vi "Install latest RSS and all addons.vi"(7 "restart automatically (T)":bool=TRUE, 8 "error in (no error)":errorcluster, 10 "Repository Location":string="\\\\uto-m34-1\\c$\\Program Files (x86)\\National Instruments\\RT Images", 11 "RT Management in":refnum<class "RT Management.lvclass">) -> (0 "error out":errorcluster, 2 "broken dependencies":T1[](array[typedef]) {"dependee"."component type" items=["standard", "hidden", "system", "unknown", "startup"]; "depender"."component type" items=["standard", "hidden", "system", "unknown", "startup"]}, 3 "RT Management out":refnum<class "RT Management.lvclass">)   [LabVIEW 2015, in "RT Management.lvlib" / "RT Management.lvclass"]
uses:
  RT Management.lvclass
  <vilib>/nisyscfg/Broken Dependency 1.2.ctl
  <vilib>/nisyscfg/Software 1.2.ctl
  <vilib>/nisyscfg/Component Type.ctl
  RT Management.lvclass/RT Management.ctl
  Get SysCfg Session.vi
  <vilib>/nisyscfg/Install Set.vi
  <vilib>/nisyscfg/nisyscfg.lvlib
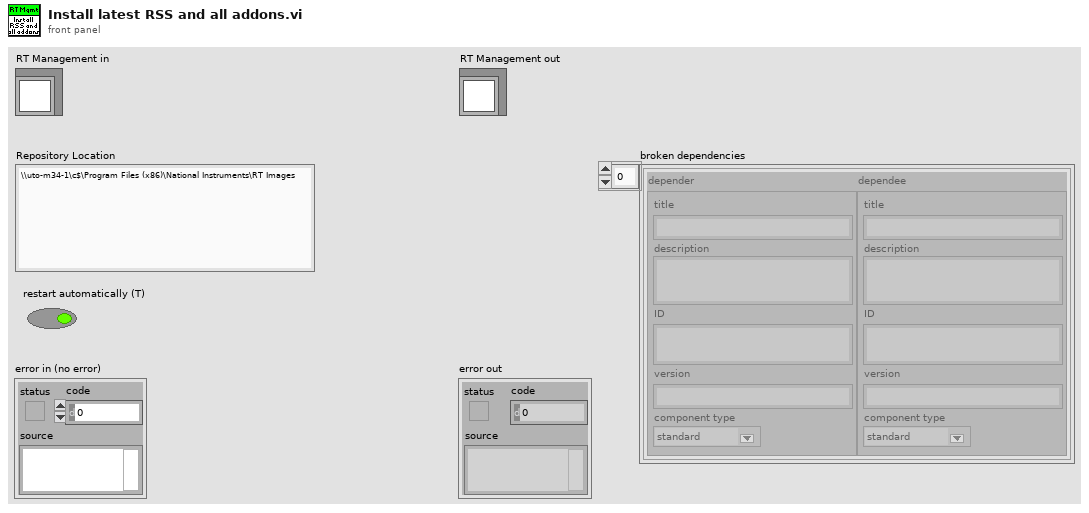
[diagram p1: front panel]
types:
  T1 = typedef "nisyscfg.lvlib/Broken Dependency 1.2.ctl" = cluster{"depender":T2, "dependee":T2}
  T2 = typedef "nisyscfg.lvlib/Software 1.2.ctl" = cluster{"title":string, "description":string, "ID":string, "version":string, "component type":T3}
  T3 = typedef "nisyscfg.lvlib/Component Type.ctl" = u32
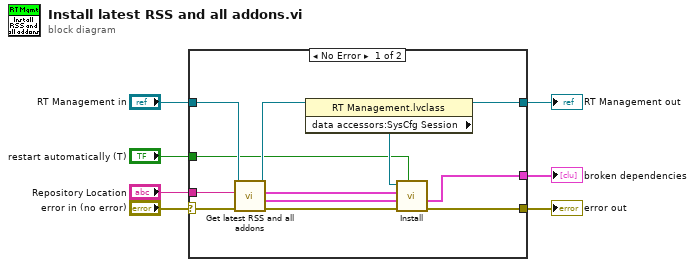
[diagram p0: block diagram]
diagram:
  n1 = case shown="No Error" "error in (no error)" {
    selector: "error in (no error)" -> [w18 w21]
    tunnel: [w19 w21] -> w6
    tunnel: [w13 w20] -> w4
    tunnel: "RT Management in" -> [w17 w20]
    tunnel: "Repository Location" -> [w10 _]
    tunnel: "restart automatically (T)" -> [w9 _]
    tunnel: [w8 _] -> w1
    frame No Error {
      n2 = call "Get latest RSS and all addons.vi"("error in (no error)"=w18, "Repository Location"=w10, "RT Management in"=w17) -> ("error out"=w16:errorcluster, "add-ons"=w12:T2[], "software set"=w11:T2, "RT Management out"=w15:refnum<class "RT Management.lvclass">)  [unwired: 4 in, 1 out]
      n3 = property class="RT Management.lvclass"(reference=w15) -> (reference out=w13:refnum<class "RT Management.lvclass">, "data accessors:SysCfg Session"=w14:refnum<k21>)  [unwired: 1 in, 1 out]
      n4 = call-poly <vilib>:"Install.vi"("Restart Automatically (T)"=w9, "error in (no error)"=w16, "Add-ons to Install"=w12, "Software Set"=w11, "Session in"=w14) -> ("error out"=w19:errorcluster, "Broken Dependencies"=w8:T1[])  [unwired: 4 in, 1 out]
    }
    frame Error {
    }
  }
  "error out" <- w6
  "RT Management out" <- w4
  "broken dependencies" <- w1
